vi "cluster2array.vi"(11 "Params":T2={"Mice ID"=[], "ExpType"=[], "Trial Interval"=[], "Pulse Duration"=[158.0, 152.0, 156.0, 167.0, 172.0], "microL_per_pulse"=[6.0, 6.0, 6.0, 6.0, 6.0], "Response Interval"=[1000.0, 1000.0, 1000.0, 1000.0, 1000.0], "Bad Delay"=[], "Response Period"=[], "liquid_type"="water", "Stimuli"=[], "Rewarded Stimuli"=[], "Air Dur"=50.0} {"Air Dur" format="%#_13g"}) -> (3 "Array":T1[](array[typedef]))   [LabVIEW 2014]
uses:
  ParamsArray.ctl
  ParamsArray2.ctl
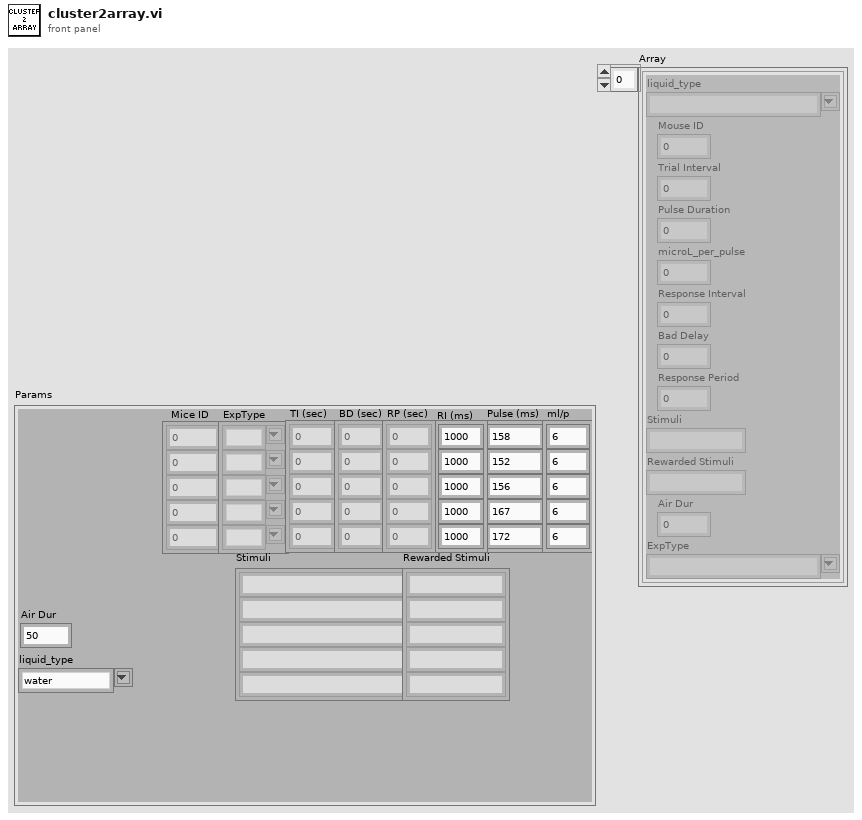
[diagram p1: front panel]
types:
  T1 = typedef "ParamsArray2.ctl" = cluster{"liquid_type":string, "Mouse ID":dbl, "Trial Interval":dbl, "Pulse Duration":dbl, "microL_per_pulse":dbl, "Response Interval":dbl, "Bad Delay":dbl, "Response Period":dbl, "Stimuli":string, "Rewarded Stimuli":string, "Air Dur":dbl, "ExpType":string}
  T2 = typedef "ParamsArray.ctl" = cluster{"Mice ID":dbl[], "ExpType":string[], "Trial Interval":dbl[], "Pulse Duration":dbl[], "microL_per_pulse":dbl[], "Response Interval":dbl[], "Bad Delay":dbl[], "Response Period":dbl[], "liquid_type":string, "Stimuli":string[], "Rewarded Stimuli":string[], "Air Dur":dbl}
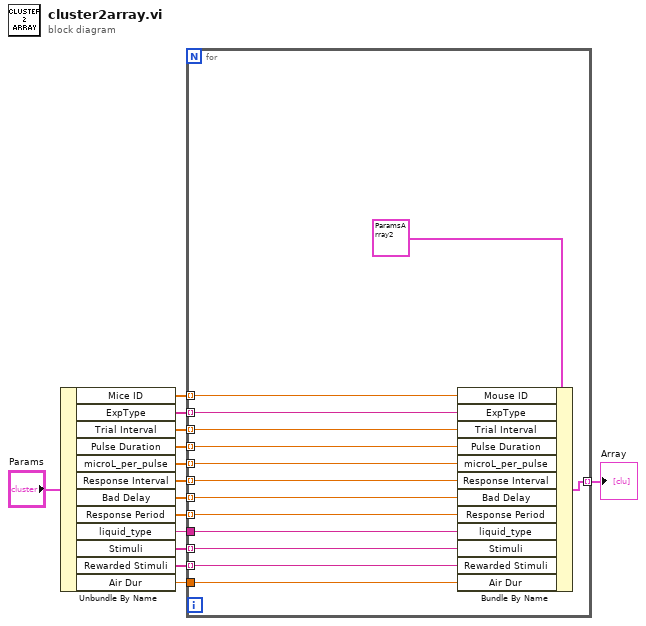
[diagram p0: block diagram]
diagram:
  n1 = Unbundle By Name("Params") -> ("Mice ID"=w14:dbl[], "ExpType"=w13:string[], "Trial Interval"=w12:dbl[], "Pulse Duration"=w5:dbl[], "microL_per_pulse"=w11:dbl[], "Response Interval"=w10:dbl[], "Bad Delay"=w9:dbl[], "Response Period"=w8:dbl[], "liquid_type"=w7:string, "Stimuli"=w6:string[], "Rewarded Stimuli"=w4:string[], "Air Dur"=w2:dbl)
  n2 = for {
    tunnel: w14 -> [w26] mode=indexing
    tunnel: w13 -> [w25] mode=indexing
    tunnel: w12 -> [w24] mode=indexing
    tunnel: w5 -> [w23] mode=indexing
    tunnel: w11 -> [w22] mode=indexing
    tunnel: w10 -> [w21] mode=indexing
    tunnel: w9 -> [w20] mode=indexing
    tunnel: w8 -> [w19] mode=indexing
    tunnel: w7 -> [w18]
    tunnel: w6 -> [w17] mode=indexing
    tunnel: w4 -> [w16] mode=indexing
    tunnel: [w28] -> w1 mode=indexing
    tunnel: w2 -> [w15]
    n3 = Bundle By Name(cluster=T1 {"liquid_type"="water", "Mouse ID"=76.0, "Trial Interval"=0.0, "Pulse Duration"=158.0, "microL_per_pulse"=6.0, "Response Interval"=1000.0, "Bad Delay"=0.0, "Response Period"=0.0, "Stimuli"="95", "Rewarded Stimuli"="95", "Air Dur"=0.0, "ExpType"=""} ("Params"), "Mouse ID"=w26, "ExpType"=w25, "Trial Interval"=w24, "Pulse Duration"=w23, "microL_per_pulse"=w22, "Response Interval"=w21, "Bad Delay"=w20, "Response Period"=w19, "liquid_type"=w18, "Stimuli"=w17, "Rewarded Stimuli"=w16, "Air Dur"=w15) -> (w28:T1)
  }
  "Array" <- w1
